vi "Create File structure.vi"(11 "Dir":string) -> (3 "created path":path)   [LabVIEW 2018]
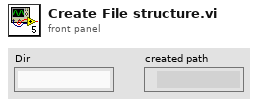
[diagram p1: front panel]
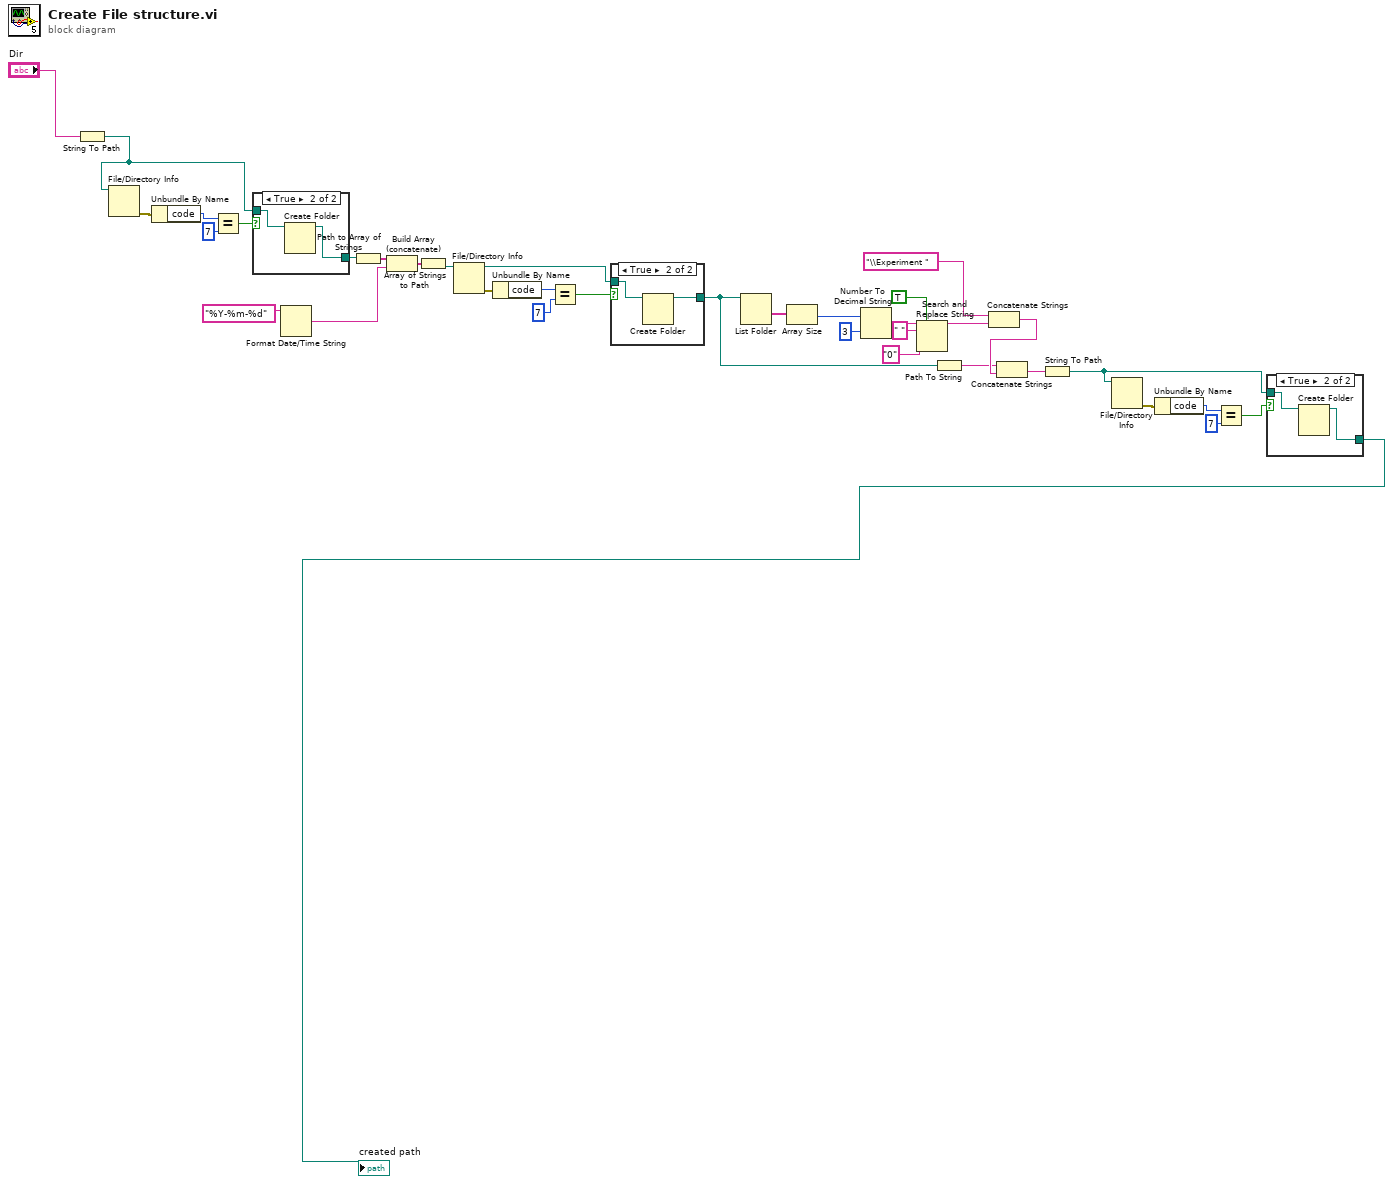
[diagram p0: block diagram]
diagram:
  n1 = String To Path(string="Dir") -> (path=w5:path)
  n2 = File/Directory Info(path=w5) -> (error out=w1:errorcluster)  [unwired: 1 in, 6 out]
  n3 = Unbundle By Name(w1) -> ("code"=w2:i32)
  n4 = Equal?(x=w2, y=7) -> (x = y?=w4:bool)
  n5 = case shown="True" w4 {
    tunnel: w5 -> [w37 w39]
    tunnel: [w37 w38] -> w7
    frame False {
    }
    frame True {
      n6 = Create Folder(path (use dialog)=w39) -> (created path=w38:path)  [unwired: 2 in, 2 out]
    }
  }
  n7 = Format Date/Time String(time format string (%c)="%Y-%m-%d") -> (date/time string=w10:string)  [unwired: 2 in]
  n8 = Path to Array of Strings(0:w7) -> (2:w9:string[])  [unwired: 1 out]
  n9 = Build Array (concatenate)(w9, w10) -> (w11:string[])
  n10 = Array of Strings to Path(0:w11) -> (2:w13:path)  [unwired: 1 in]
  n11 = File/Directory Info(path=w13) -> (path out=w17:path, error out=w14:errorcluster)  [unwired: 1 in, 5 out]
  n12 = Unbundle By Name(w14) -> ("code"=w15:i32)
  n13 = Equal?(x=w15, y=7) -> (x = y?=w16:bool)
  n14 = case shown="True" w16 {
    tunnel: w17 -> [w40 w42]
    tunnel: [w40 w41] -> w31
    frame False {
    }
    frame True {
      n15 = Create Folder(path (use dialog)=w42) -> (created path=w41:path)  [unwired: 2 in, 2 out]
    }
  }
  n16 = List Folder(path=w31) -> (folder names=w18:string[])  [unwired: 3 in, 3 out]
  n17 = Array Size(array=w18) -> (size(s)=w19:i32)
  n18 = Number To Decimal String(number=w19, width (-)=i16 3) -> (decimal integer string=w21:string)
  n19 = Search and Replace String(replace all?=TRUE ("replace all? (F)"), input string=w21, search string=" ", replace string="0" ("replace string (\"\")")) -> (result string=w25:string)  [unwired: 4 in, 3 out]
  n20 = Path To String(path=w31) -> (string=w30:string)
  n21 = Concatenate Strings("\\Experiment " ("string"), w25) -> (w32:string)
  n22 = Concatenate Strings(w30, w32) -> (w33:string)
  n23 = String To Path(string=w33) -> (path=w34:path)
  n24 = File/Directory Info(path=w34) -> (error out=w27:errorcluster)  [unwired: 1 in, 6 out]
  n25 = Unbundle By Name(w27) -> ("code"=w28:i32)
  n26 = Equal?(x=w28, y=7) -> (x = y?=w35:bool)
  n27 = case shown="True" w35 {
    tunnel: w34 -> [w43 w45]
    tunnel: [w43 w44] -> w36
    frame False {
    }
    frame True {
      n28 = Create Folder(path (use dialog)=w45) -> (created path=w44:path)  [unwired: 2 in, 2 out]
    }
  }
  "created path" <- w36
